vi "redirect to another spartan cgi.vi"(8 "error in (no error)":errorcluster, 9 "query params":T1, 10 "New URL (/cgi-bin/testing.vit)":string="/cgi-bin/testing.vit", 11 "Original Header In (to be replaced)":string) -> (0 "error out":errorcluster, 3 "Redirection Header":string)   [LabVIEW 2011]
uses:
  ITK EXT/utils/keyedarr.llb/Keyed Array.ctl
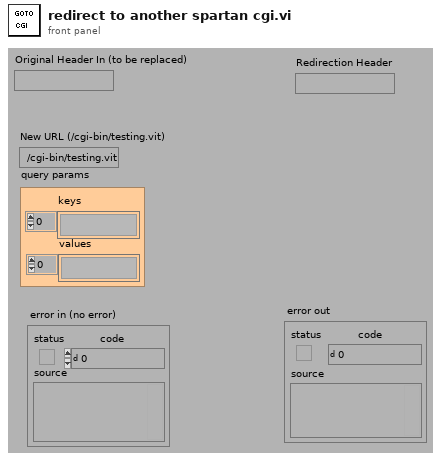
[diagram p1: front panel]
types:
  T1 = typedef "Keyed Array.ctl" = cluster{"keys":string[], "values":string[]}
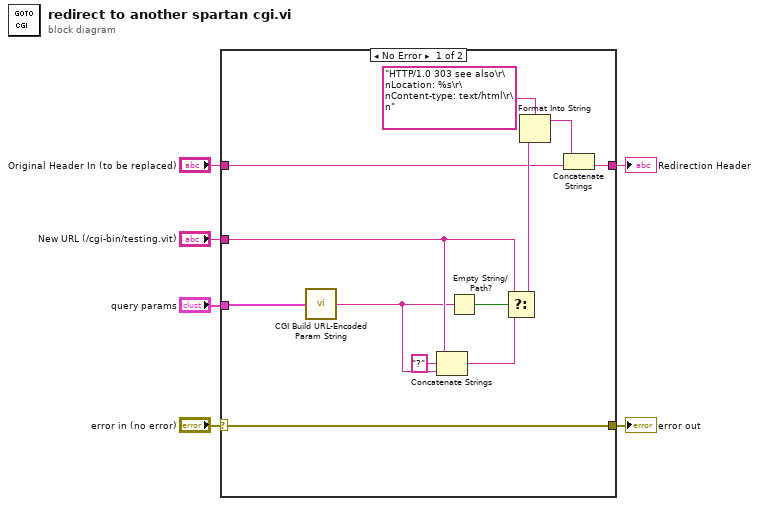
[diagram p0: block diagram]
diagram:
  n1 = case shown="No Error" "error in (no error)" {
    selector: "error in (no error)" -> [w12 w19]
    tunnel: [w7 w20] -> w6
    tunnel: "New URL (/cgi-bin/testing.vit)" -> [w16 _]
    tunnel: [w12 w19] -> w3
    tunnel: "Original Header In (to be replaced)" -> [w8 w20]
    tunnel: "query params" -> [w11 _]
    frame No Error {
      n2 = call "CGI Build URL-Encoded Param String.vi"("params"=w11) -> ("url-encoded param string"=w10:string)
      n3 = Concatenate Strings(w16, "?" ("string"), w10) -> (w14:string)
      n4 = Empty String/Path?(string/path=w10) -> (empty?=w17:bool)
      n5 = Select(t=w16, s=w17, f=w14) -> (s? t:f=w15:string)
      n6 = Format Into String(format string="HTTP/1.0 303 see also\r\nLocation: %s\r\nContent-type: text/html\r\n", w15) -> (resulting string=w9:string)  [unwired: 2 in, 1 out]
      n7 = Concatenate Strings(w9, w8) -> (w7:string)
    }
    frame Error {
    }
  }
  "Redirection Header" <- w6
  "error out" <- w3
